vi "setFrameSize.vi"(8 "error":errorcluster, 10 "FrameSize [40|48|60|72]":u8, 11 "connection ID":refnum<k5>) -> (0 "error out":errorcluster, 3 "connection ID out":refnum<k5>)   [LabVIEW 2016, in "AMC_VIs.lvlib"]
doc: "This function reads the frequency for the sensor read out of the RES position on a specific axis\nInputs:\n -- connection string (from connect_TCP.vi)\n -- FrameSize [40,48,60,72]\n\nOutputs:\n -- connection ID out"
uses:
  AMC_VIs.lvlib
panel:
  out "JSON-response":string="{\"jsonrpc\":\"2.0\",\"method\":\"\",\"params\":[5,1.245,true,\"name\"],\"id\":\"1\"}"
  out "JSON request":string
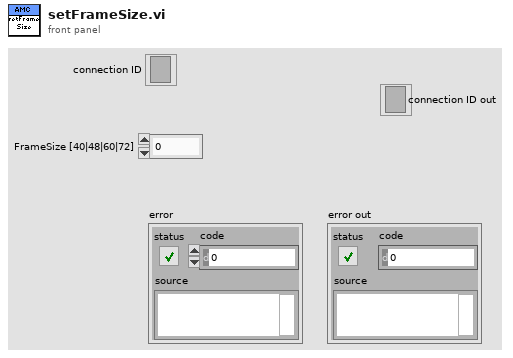
[diagram p1: front panel]
types:
  T1 = cluster{"jsonrpc":string, "method":string, "params":i32[], "id":string, "api":string}
  T2 = cluster{"jsonrpc":string, "result":i32[], "id":string}
  T3 = enum16{"Standard", "Buffered", "CRLF", "Immediate"}
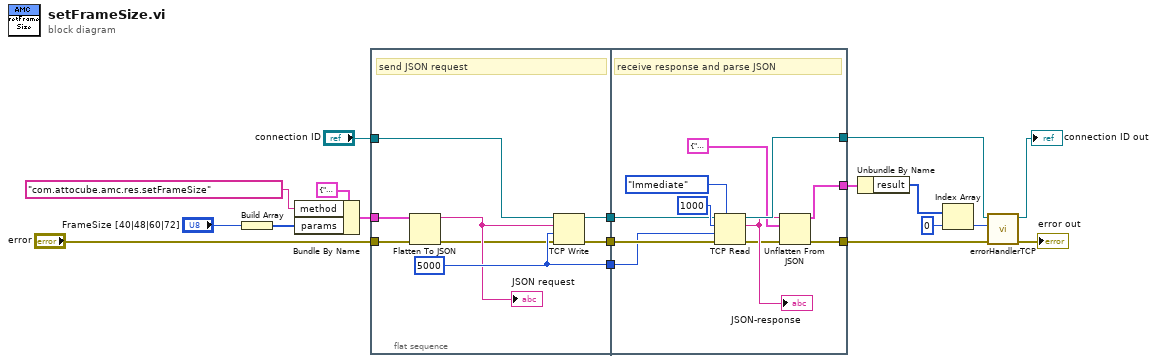
[diagram p0: block diagram]
diagram:
  n1 = Build Array("FrameSize [40|48|60|72]") -> (w11:u8[])
  n2 = Bundle By Name(cluster=T1 {"jsonrpc"="2.0", "method"="com.attocube.amc.res.setRESReadOutFreq", "params"=[0, 2712], "id"="1", "api"="2"} ("InputParams 2"), "method"="com.attocube.amc.res.setFrameSize", "params"=w11) -> (w10:T1)
  n3 = flat-sequence {
    tunnel: "connection ID" -> [w26]
    tunnel: [w24] -> w18
    tunnel: [w25] -> w17
    tunnel: "error" -> [w20]
    tunnel: [w23] -> w16
    tunnel: w10 -> [w22]
    tunnel: [w33] -> w3
    tunnel: w18 -> [w35]
    tunnel: w17 -> [w34]
    tunnel: [w29] -> w6
    tunnel: w16 -> [w32]
    tunnel: [w28] -> w9
    frame #0 {
      w23 = 5000 ("timeout ms (25000)")
      # "send JSON request"
      n4 = Flatten To JSON(anything=w22, error in (no error)=w20) -> (JSON string=w21:string, 11:w19:errorcluster)  [unwired: 1 in]
      "JSON request" <- w21
      n5 = TCP Write(connection ID=w26, data in=w21, error in (no error)=w19, 9:w23) -> (connection ID out=w24:refnum<k5>, error out=w25:errorcluster)  [unwired: 1 out]
    }
    frame #1 {
      # "receive response and parse JSON"
      n6 = TCP Read(connection ID=w35, bytes to read=1000, error in (no error)=w34, 7:T3."Immediate" ("mode (standard)"), 9:w32) -> (connection ID out=w33:refnum<k5>, data out=w31:string, error out=w30:errorcluster)
      "JSON-response" <- w31
      n7 = Unflatten From JSON(JSON string=w31, type and defaults=T2 {"jsonrpc"="2.0", "result"=[0, 2712], "id"="1"} ("InputParams 2"), error in (no error)=w30) -> (value=w28:T2, error out=w29:errorcluster)  [unwired: 4 in]
    }
  }
  n8 = Unbundle By Name(w9) -> ("result"=w7:i32[])
  n9 = Index Array(array=w7, index=0) -> (element=w5:i32)
  n10 = call "errorHandlerTCP.vi"("error in"=w6, "error number"=w5, "connection ID"=w3) -> ("error out"=→"error out":errorcluster, "connection ID"=→"connection ID out":refnum<k5>)  [unwired: 7 in]
